vi "Build Config Maps.vi"(8 "error in (no error)":errorcluster, 11 "VolatusConfig in":refnum<class "VolatusConfig.lvclass">) -> (0 "error out":errorcluster, 3 "VolatusConfig out":refnum<class "VolatusConfig.lvclass">)   [LabVIEW 2020, in "VolatusConfig.lvlib" / "VolatusConfig.lvclass"]
uses:
  VolatusConfig.lvclass
  VolatusConfig.lvclass/VolatusConfig.ctl
  VolatusConfig.lvlib
  lv-cdm/CDM-Config/Config Manager/Config Manager.lvclass
  Meta Type.ctl
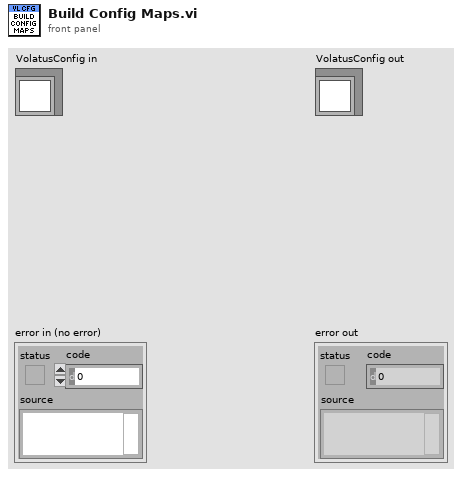
[diagram p1: front panel]
types:
  T1 = typedef "VolatusConfig.lvlib/Meta Type.ctl" = enum16{"VL_System", "VL_Cluster", "VL_Node", "VL_Task"}
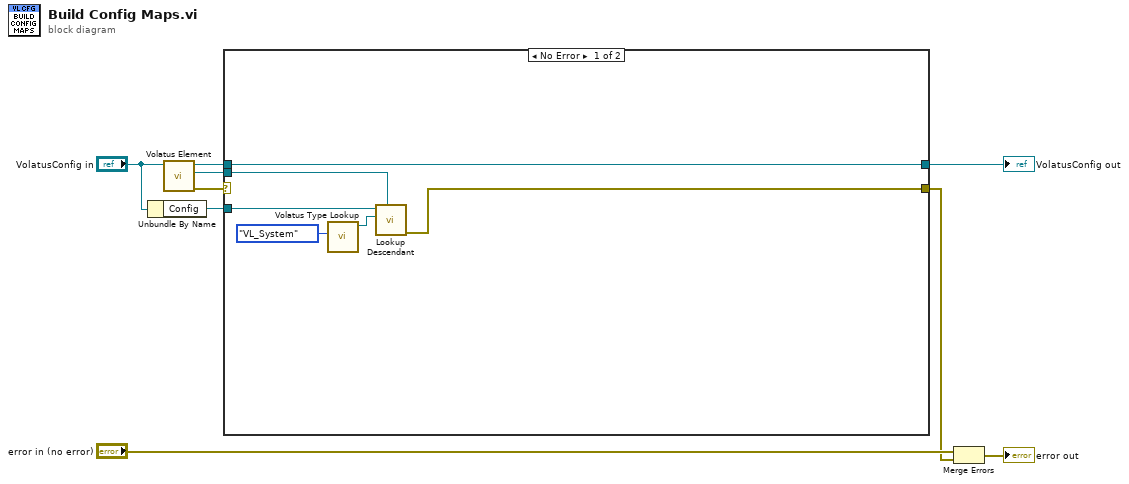
[diagram p0: block diagram]
diagram:
  n1 = Unbundle By Name("VolatusConfig in") -> ("Config"=w1:refnum<class "Config Manager.lvclass">)
  n2 = call "Volatus Element.vi"("VolatusConfig in"="VolatusConfig in") -> ("error out"=w4:errorcluster, "Volatus Element"=w3:refnum<class "Config Element.lvclass">, "VolatusConfig out"=w5:refnum<class "VolatusConfig.lvclass">)  [unwired: 8 in]
  n3 = case shown="No Error" w4 {
    selector: w4 -> [_ w16]
    tunnel: w5 -> [w11 w17]
    tunnel: [w11 w17] -> w8
    tunnel: [w10 w16] -> w6
    tunnel: w3 -> [w14 _]
    tunnel: w1 -> [w15 _]
    frame No Error {
      n4 = call "Volatus Type Lookup.vi"("Meta Type"=Meta_Type."VL_System") -> ("Config Lookup out"=w12:refnum<class "Config Lookup.lvclass">)  [unwired: 9 in, 1 out]
      n5 = call "Lookup Descendant.vi"("Start (Root)"=w14, "Lookup"=w12, "Config Manager in"=w15) -> ("error out"=w10:errorcluster)  [unwired: 6 in, 2 out]
    }
    frame Error {
    }
  }
  "VolatusConfig out" <- w8
  n6 = Merge Errors("error in (no error)", w6) -> (→"error out":errorcluster)
